vi "Update Status.vi"(10 "error in (no error)":errorcluster, 11 "Status Bar Text":string) -> (2 "error out":errorcluster)   [LabVIEW 2020, in "RxnRover.lvlib"]
uses:
  RxnRover.lvlib
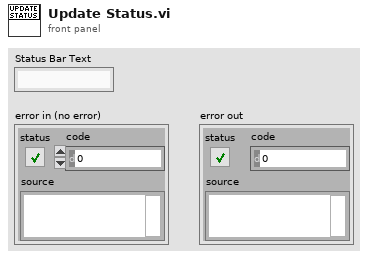
[diagram p1: front panel]
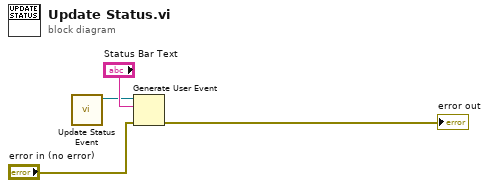
[diagram p0: block diagram]
diagram:
  n1 = call "Update Status Event.vi"() -> ("Update Status"=w1:refnum<user-event>)  [unwired: 11 in]
  n2 = Generate User Event(user event=w1, event data cluster="Status Bar Text", error in="error in (no error)") -> (error out=→"error out":errorcluster)  [unwired: 1 in, 1 out]
